vi "ATF-Pump-DO waveform Samples bulider.vi"(7 "Samples 2":i32=10, 9 "Data input 2":waveform(dbl)[](array[waveform]), 11 "DO_Data RD":refnum<queue>) -> (1 "Array 4":timestamp[][](array[timestamp]), 2 "Array 3":dbl[][](array[numeric]))   [LabVIEW 2022 SP3]
panel:
  in  "Data input 3":waveform(dbl)[](array[waveform])
  out "Data out 2":waveform(dbl)[](array[waveform])
  out "overflow? 2":bool
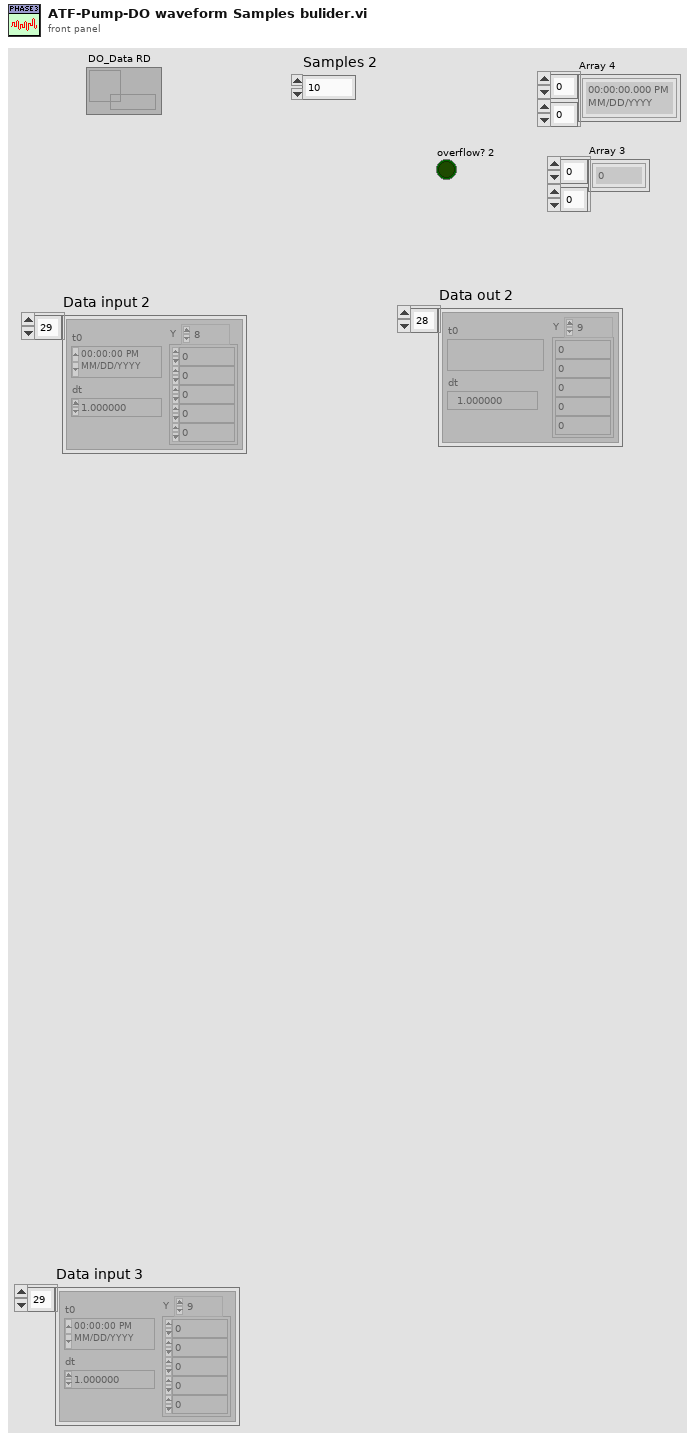
[diagram p1: front panel]
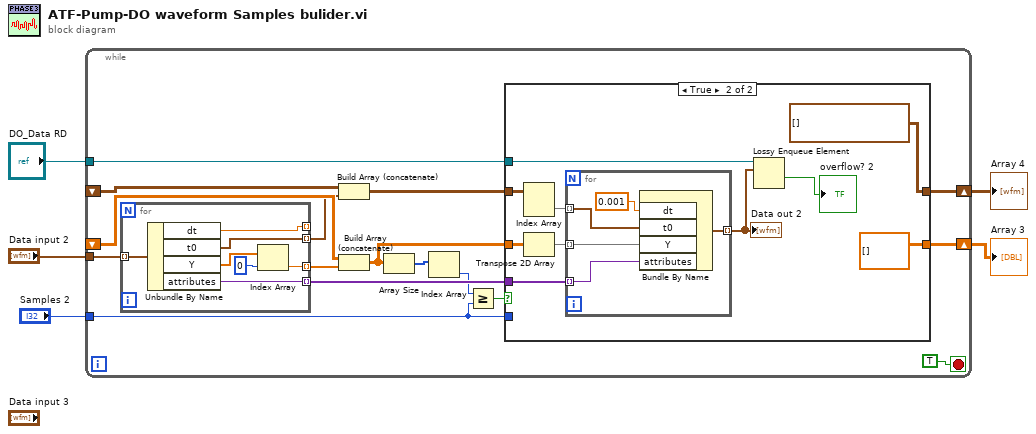
[diagram p0: block diagram]
diagram:
  n1 = while {
    tunnel: "Data input 2" -> [w17]
    tunnel: "Samples 2" -> [w16]
    tunnel: "DO_Data RD" -> [w15]
    shift-right: [w18] -> w4
    shift-left: _ -> [w21]
    shift-right: [w19] -> w5
    shift-left: _ -> [w20]
    stop <- TRUE stop-if-true
    n2 = for {
      tunnel: w17 -> [w45] mode=indexing
      tunnel: [w43] -> w6 mode=indexing
      tunnel: [w41] -> w11 mode=indexing
      tunnel: [w40] -> w13 mode=indexing
      tunnel: [w39] -> _ mode=indexing
      n3 = Unbundle By Name(w45) -> ("dt"=w39:dbl, "t0"=w41:timestamp, "Y"=w44:dbl[], "attributes"=w40:variant)
      n4 = Index Array(array=w44, index=0) -> (element=w43:dbl)
    }
    n5 = Build Array (concatenate)(w20, w11) -> (w12:timestamp[][])
    n6 = Build Array (concatenate)(w21, w6) -> (w9:dbl[][])
    n7 = Array Size(array=w9) -> (size(s)=w7:i32[])
    n8 = Index Array(array=w7) -> (element=w8:i32)  [unwired: 1 in]
    n9 = Greater Or Equal?(x=w8, y=w16) -> (x >= y?=w10:bool)
    n10 = case shown="True" w10 {
      tunnel: w9 -> [w23 w28]
      tunnel: [w23 dbl[][] []] -> w18
      tunnel: w12 -> [w22 w25]
      tunnel: [w22 timestamp[][] []] -> w19
      tunnel: w13 -> [_ w33]
      tunnel: w16 -> [_ _]
      tunnel: w15 -> [_ w31]
      frame False {
      }
      frame True {
        n11 = Index Array(array=w25) -> (element=w24:timestamp[])  [unwired: 2 in]
        n12 = Transpose 2D Array(2D array=w28) -> (transposed array=w32:dbl[][])
        n13 = for {
          tunnel: w32 -> [w38] mode=indexing
          tunnel: w33 -> [w37] mode=indexing
          tunnel: [w36] -> w30 mode=indexing
          tunnel: w24 -> [w35] mode=indexing
          n14 = Bundle By Name("dt"=0.001, "t0"=w35, "Y"=w38, "attributes"=w37) -> (w36:waveform(dbl))  [unwired: 1 in]
        }
        "Data out 2" <- w30
        n15 = Lossy Enqueue Element(queue=w31, element=w30) -> (overflow?=→"overflow? 2":bool)  [unwired: 1 in, 3 out]
      }
    }
  }
  "Array 4" <- w5
  "Array 3" <- w4
